vi "WILT Agilent Switch Setup.vi"(8 "Error In":errorcluster, 11 "VISA Resource Name":refnum<visa-resource-name>="GPIB0::9::INSTR") -> (0 "Error Out":errorcluster)   [LabVIEW 2016]
uses:
  Drivers/Agilent 34972/Agilent 34970.lvlib
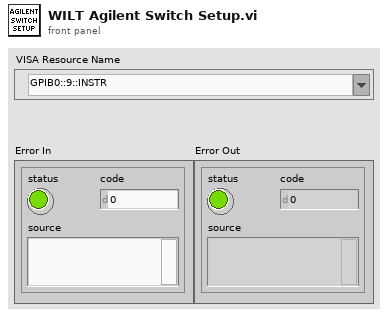
[diagram p1: front panel]
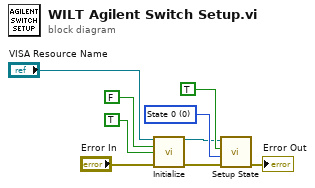
[diagram p0: block diagram]
diagram:
  w8 = u16 0 items=["State 0", "State 1", "State 2", "State 3", "State 4", "State 5", "Preset State"] ("Setup State (6:Preset)")
  n1 = call "Initialize.vi"("VISA Resource Name"="VISA Resource Name", "ID Query (T: Check)"=FALSE, "Reset (T: Reset)"=TRUE, "error in (no error)"="Error In") -> ("VISA Resource Name Out"=w3:refnum<visa-resource-name>, "error out"=w9:errorcluster)  [unwired: 10 in]
  n2 = call "Setup State.vi"("error in (no error)"=w9, "Setup State (6:Preset)"=w8, "Recall/Save (F=Recall)"=TRUE, "VISA Resource Name"=w3) -> ("error out"=→"Error Out":errorcluster)  [unwired: 6 in, 1 out]
